vi "Speed PI Control.vi"() -> ()   [LabVIEW 2016]
panel:
  in  "Slide":dbl(slide) min=0.0 max=5.0 step=0.1 scale=0.0..10.0
  in  "I-Gain":dbl(slide)=1.0 scale=0.0..2.0
  in  "P-Gain":dbl(slide)=1.0 scale=0.0..2.0
  in  "Setpoint Speed (rps)":dbl(slide) scale=-8.3..8.3
  out "Speed (rps)":dynamicdata(graph)
  in  "stop (F)":bool
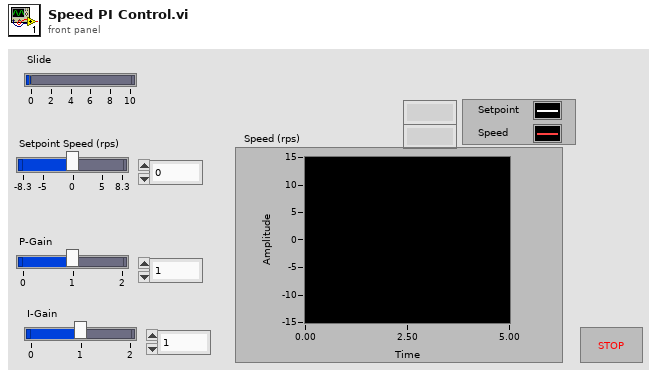
[diagram p1: front panel]
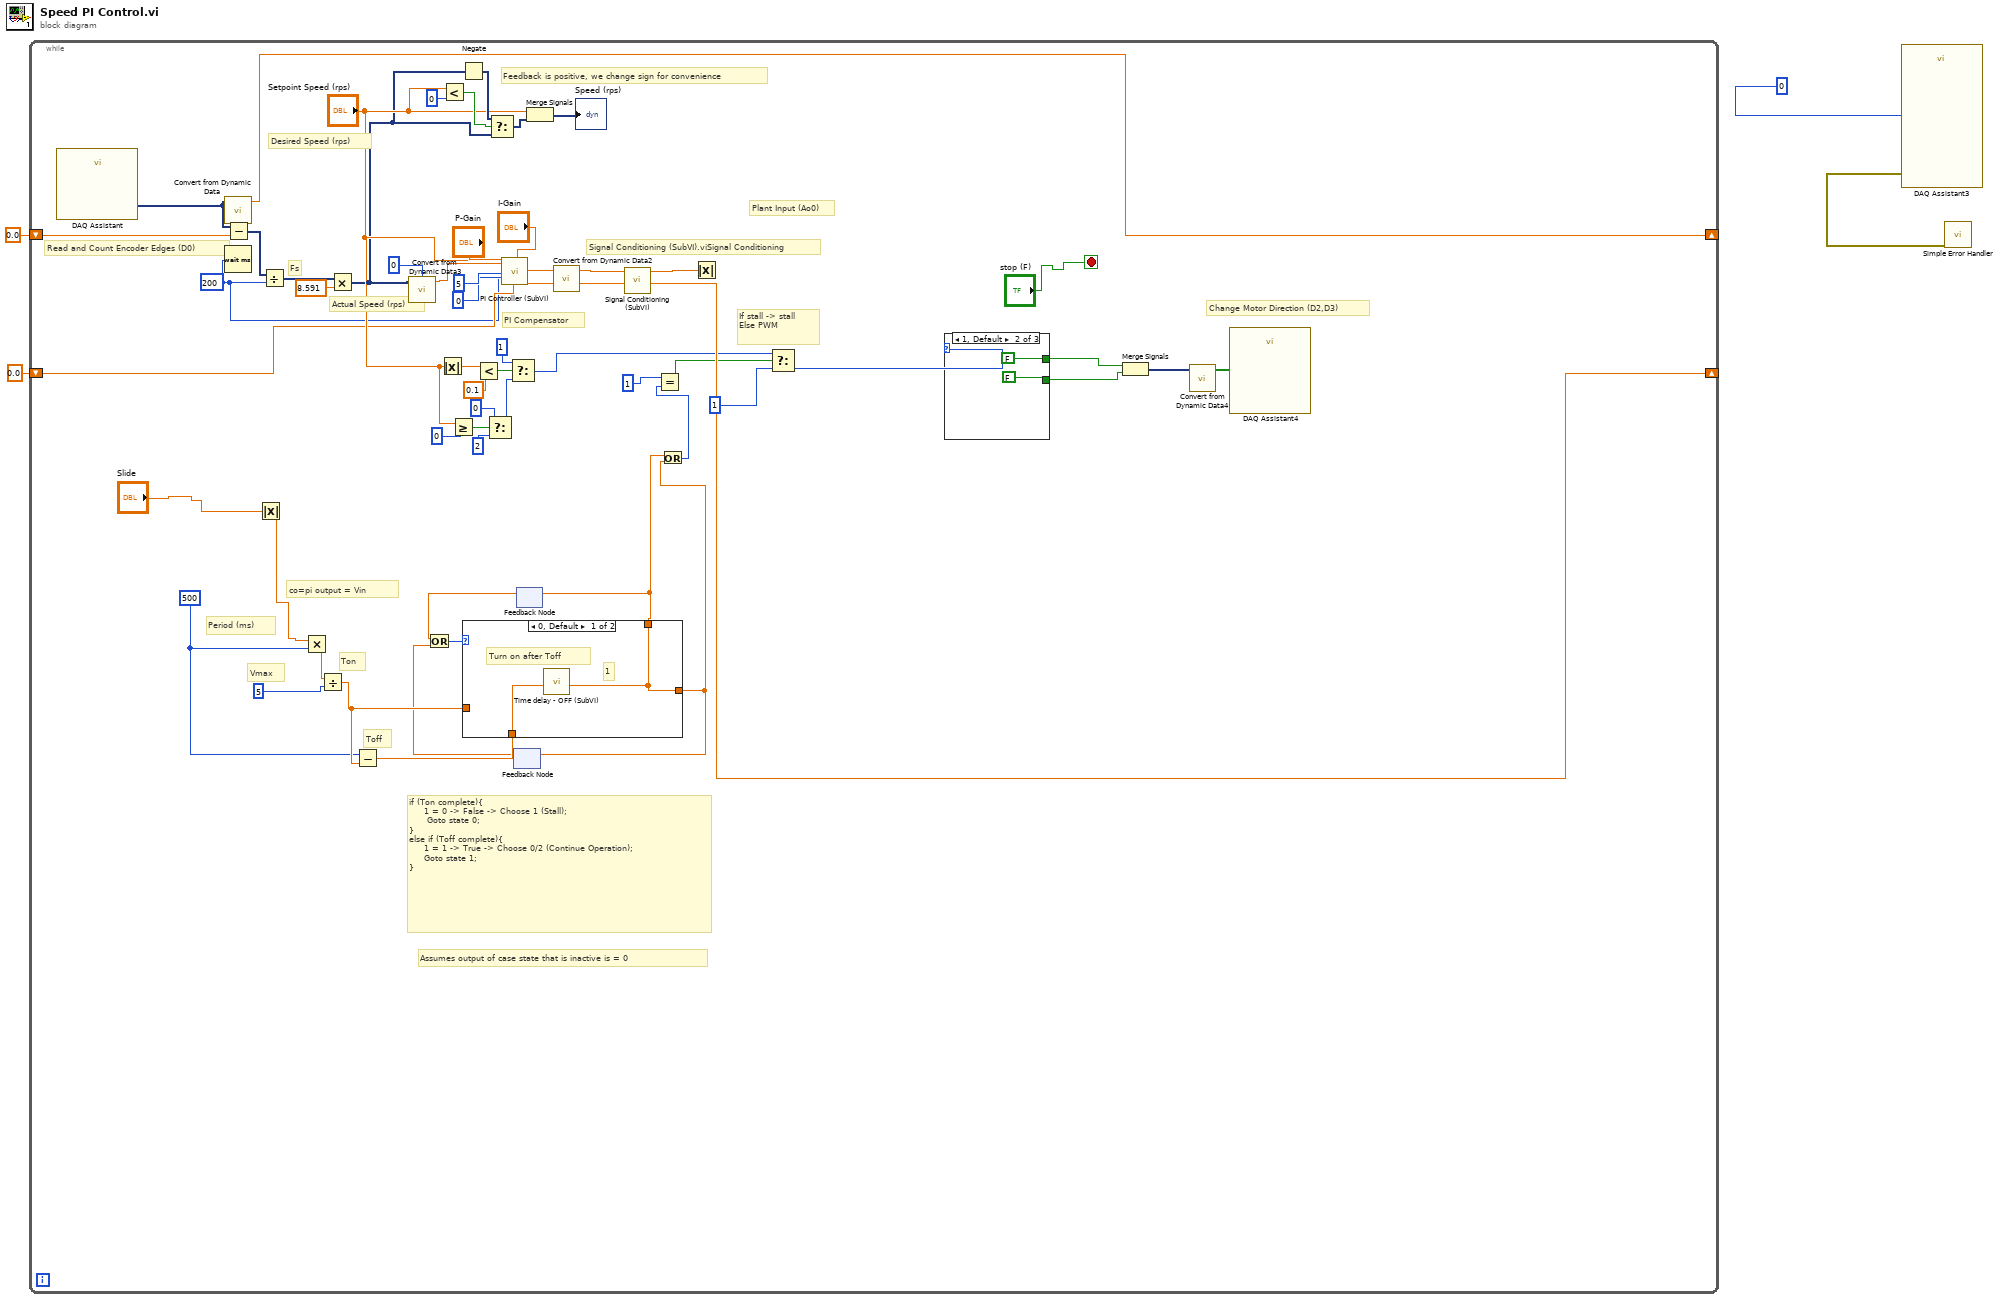
[diagram p0: block diagram]
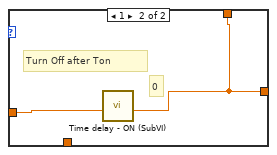
[diagram p2: hidden frame]
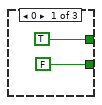
[diagram p3: hidden frame]
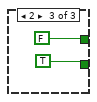
[diagram p4: hidden frame]
diagram:
  n1 = while {
    shift-right: [w61] -> _
    shift-left: 0.0 -> [w60]
    shift-right: [w31] -> _
    shift-left: 0.0 -> [w34]
    stop <- "stop (F)" stop-if-true
    w15 = 500
    w33 = 200
    # "Assumes output of case state that is inactive is = 0"
    # "if (Ton complete){\n     1 = 0 -> False -> Choose 1 (Stall);\n      Goto state 0;\n}\nelse if (Toff complete){\n     1 = 1 -> True -> Choose 0/2 (Continue Operation);\n     Goto state 1;\n}"
    # "Toff"
    # "Change Motor Direction (D2,D3)"
    # "If stall -> stall\nElse PWM"
    # "Ton"
    # "Vmax"
    # "co=pi output = Vin"
    # "Period (ms)"
    # "Desired Speed (rps)"
    # "Feedback is positive, we change sign for convenience"
    # "Signal Conditioning (SubVI).viSignal Conditioning"
    # "PI Compensator"
    # "Fs"
    # "Actual Speed (rps)"
    # "Read and Count Encoder Edges (D0)"
    # "Plant Input (Ao0)"
    n2 = call "DAQ Assistant"() -> ("data"=w56:dynamicdata)  [unwired: 16 in, 3 out]
    n3 = call "Convert from Dynamic Data"("Dynamic Data Type"=w56) -> ("Scalar"=w61:dbl)  [unwired: 3 in]
    n4 = Wait (ms)(milliseconds to wait=w33) -> ()  [unwired: 1 out]
    n5 = Subtract(x=w56, y=w60) -> (x-y=w59:dynamicdata)
    n6 = Absolute Value(x="Slide") -> (abs(x)=w25:dbl)
    n7 = Divide(x=w59, y=w33) -> (x/y=w58:dynamicdata)
    n8 = Multiply(x=w25, y=w15) -> (x*y=w29:dbl)
    n9 = Divide(x=w29, y=5) -> (x/y=w16:dbl)
    n10 = Multiply(x=w58, y=8.591) -> (x*y=w32:dynamicdata)
    n11 = Subtract(x=w15, y=w16) -> (x-y=w14:dbl)
    n12 = call "Convert from Dynamic Data3"("Dynamic Data Type"=w32, "Channel"=0) -> ("Scalar"=w39:dbl)  [unwired: 2 in]
    n13 = Absolute Value(x="Setpoint Speed (rps)") -> (abs(x)=w50:dbl)
    n14 = Less?(x="Setpoint Speed (rps)", y=0) -> (x < y?=w42:bool)
    n15 = Greater Or Equal?(x="Setpoint Speed (rps)", y=0) -> (x >= y?=w53:bool)
    n16 = Negate(x=w32) -> (-x=w41:dynamicdata)
    n17 = Less?(x=w50, y=0.1) -> (x < y?=w48:bool)
    n18 = Select(t=0, s=w53, f=2) -> (s? t:f=w47:i32)
    n19 = Select(t=w41, s=w42, f=w32) -> (s? t:f=w43:dynamicdata)
    n20 = call "PI Controller (SubVI).vi"("sp"="Setpoint Speed (rps)", "pv"=w39, "maxim"=5, "minim"=0, "p"="P-Gain", "errsum"=w34, "i"="I-Gain", "h"=w33) -> ("output variable"=w30:dbl, "errsum"=w31:dbl)  [unwired: 18 in]
    n21 = Select(t=1, s=w48, f=w47) -> (s? t:f=w24:i32)
    n22 = feedback #1() -> (w11:dbl)  [unwired: 1 in]
    n23 = feedback #2() -> (w12:dbl)  [unwired: 1 in]
    n24 = Or(x=w12, y=w11) -> (x .or. y?=w13:i32)
    n25 = case shown="0, Default" w13 {
      tunnel: w16 -> [_ w65]
      tunnel: [w62 w64] -> w10
      tunnel: w14 -> [w63 _]
      tunnel: [w62 w64] -> w9
      frame 0, Default {
        # "1"
        # "Turn on after Toff"
        n26 = call "Time delay - OFF (SubVI).vi"("Toff"=w63) -> ("Output"=w62:dbl)  [unwired: 8 in]
      }
      frame 1 {
        # "Turn Off after Ton"
        # "0"
        n27 = call "Time delay - ON (SubVI).vi"("Ton"=w65) -> ("Output"=w64:dbl)  [unwired: 8 in]
      }
    }
    n28 = feedback-in #1(w10) -> ()
    n29 = feedback-in #2(w9) -> ()
    n30 = Merge Signals("Setpoint Speed (rps)", w43) -> (→"Speed (rps)":dynamicdata)
    n31 = call "Convert from Dynamic Data2"("Dynamic Data Type"=w30) -> ("Scalar"=w6:dbl)  [unwired: 3 in]
    n32 = call "Signal Conditioning (SubVI).vi"("Input"=w6) -> ("Output"=w46:dbl)  [unwired: 10 in]
    n33 = Or(x=w9, y=w10) -> (x .or. y?=w8:i32)
    n34 = Equal?(x=1, y=w8) -> (x = y?=w18:bool)
    n35 = Absolute Value(x=w46) -> ()  [unwired: 1 out]
    n36 = Select(t=w24, s=w18, f=1) -> (s? t:f=w19:i32)
    n37 = case shown="1, Default" w19 {
      tunnel: [TRUE FALSE FALSE] -> w21
      tunnel: [FALSE FALSE TRUE] -> w20
      frame 0 {
      }
      frame 1, Default {
      }
      frame 2 {
      }
    }
    n38 = Merge Signals(w21, w20) -> (w23:dynamicdata)
    n39 = call "Convert from Dynamic Data4"("Dynamic Data Type"=w23) -> ("Array"=w22:bool[])  [unwired: 3 in]
    n40 = call "DAQ Assistant4"("data"=w22) -> ()  [unwired: 17 in, 2 out]
  }
  n41 = call "DAQ Assistant3"("data"=0) -> ("error out"=w2:errorcluster)  [unwired: 17 in, 1 out]
  n42 = call <vilib>:"Simple Error Handler.vi"("error in (no error)"=w2) -> ()  [unwired: 4 in, 5 out]
